vi "Error Query.vi"(8 "error in (no error)":errorcluster, 11 "VISA resource name":refnum<visa-resource-name>) -> (0 "error out":errorcluster, 1 "Error Message":string, 2 "Error Code":i32[](array[numeric]), 3 "VISA resource name out":refnum<visa-resource-name>)   [LabVIEW 2019, in "Agilent E363X Series.lvlib"]
doc: "Queries the instrument for any errors in the instrument's error queue. It will continue to read errors until all errors have been read from the instrument. Any errors will be returned in the Error Out cluster.\n\n<B>Note:</B>\nThis VI is called automatically by most driver VIs so it is not usually necessary to call this in an application."
uses:
  Agilent E363X Series.lvlib
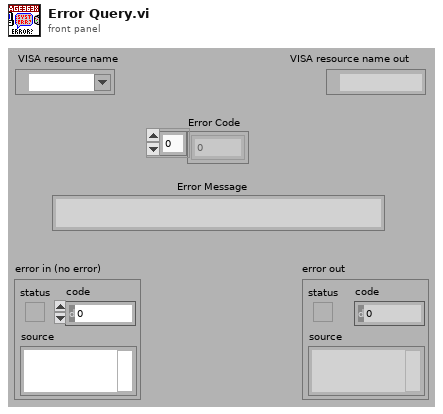
[diagram p1: front panel]
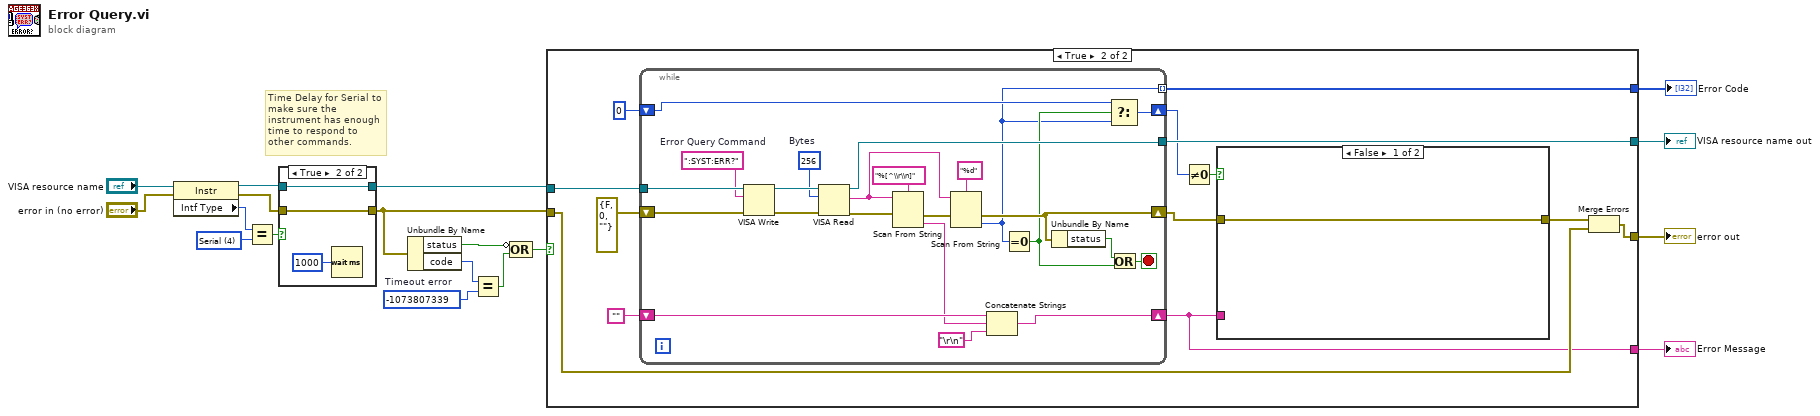
[diagram p0: block diagram]
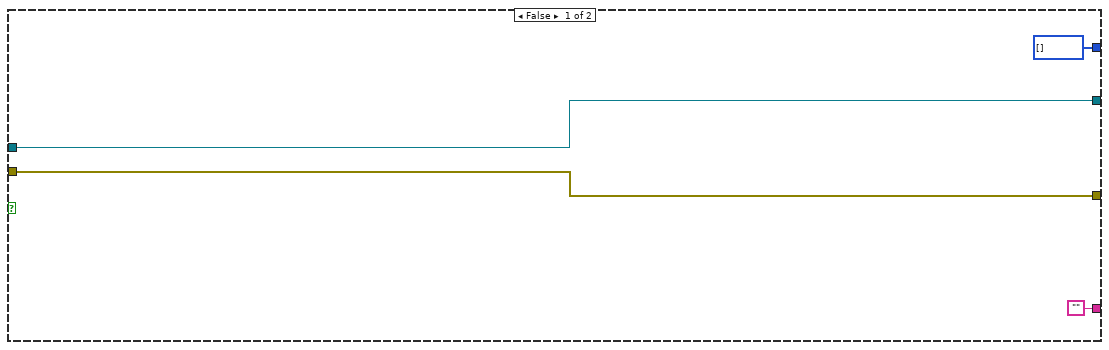
[diagram p3: hidden frame]
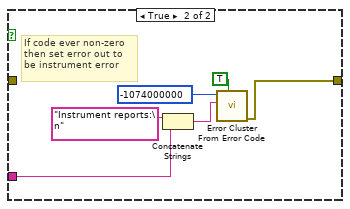
[diagram p4: hidden frame]
diagram:
  w2 = u16 4 items=["GPIB"=1, "VXI"=2, "GPIB-VXI"=3, "Serial"=4, "PXI"=5, "TCPIP"=6, "USB"=7] ("Interface Information:Interface Type")
  w15 = -1073807339  # Timeout error
  # "Time Delay for Serial to make sure the instrument has enough time to respond to other commands."
  n1 = property class="Instr"(reference="VISA resource name", error in="error in (no error)") -> (reference out=w5:refnum<visa-resource-name>, error out=w4:errorcluster, "Intf Type"=w3:u16)
  n2 = Equal?(x=w3, y=w2) -> (x = y?=w1:bool)
  n3 = case shown="True" w1 {
    tunnel: w4 -> [w19 w22]
    tunnel: [w19 w22] -> w9
    tunnel: w5 -> [w20 w21]
    tunnel: [w20 w21] -> w8
    frame False {
    }
    frame True {
      n4 = Wait (ms)(milliseconds to wait=u32 1000) -> ()  [unwired: 1 out]
    }
  }
  n5 = Unbundle By Name(w9) -> ("status"=w16:bool, "code"=w13:i32)
  n6 = Equal?(x=w13, y=w15) -> (x = y?=w14:bool)
  n7 = Compound Arithmetic op=OR(invert w16, w14) -> (w12:bool)
  n8 = case shown="True" w12 {
    tunnel: [w27 w40] -> w18
    tunnel: w8 -> [w27 w39]
    tunnel: w9 -> [w26 w33]
    tunnel: [w26 w37] -> w17
    tunnel: ["" w30] -> w11
    tunnel: [i32[] [] w29] -> w10
    frame False {
    }
    frame True {
      n9 = while {
        tunnel: [w70] -> w40
        tunnel: w39 -> [w69]
        shift-right: [w57] -> w30
        shift-left: "" -> [w60]
        shift-right: [w55] -> w31
        shift-left: 0 -> [w56]
        shift-right: [w53] -> w28
        shift-left: errorcluster {"status"=FALSE, "code"=0, "source"=""} ("error in (no error)") -> [w54]
        tunnel: [w48] -> w29 mode=indexing
        stop <- w63 stop-if-true
        w67 = u32 256  # Bytes
        w65 = ":SYST:ERR?"  # Error Query Command
        n10 = VISA Write(VISA resource name=w69, write buffer=w65, error in (no error)=w54) -> (VISA resource name out=w68:refnum<visa-resource-name>, error out=w66:errorcluster)  [unwired: 1 out]
        n11 = VISA Read(VISA resource name=w68, byte count=w67, error in (no error)=w66) -> (VISA resource name out=w70:refnum<visa-resource-name>, read buffer=w61:string, error out=w52:errorcluster)  [unwired: 1 out]
        n12 = Scan From String(format string="%[^\\r\\n]", input string=w61, error in=w52) -> (error out=w51:errorcluster, output 1=w58:string)  [unwired: 2 in, 2 out]
        n13 = Scan From String(format string="%d", input string=w61, error in=w51) -> (error out=w53:errorcluster, output 1=w48:i32)  [unwired: 2 in, 2 out]
        n14 = Concatenate Strings(w60, w58, "\r\n") -> (w57:string)
        n15 = Equal To 0?(x=w48) -> (x = 0?=w49:bool)
        n16 = Unbundle By Name(w53) -> ("status"=w50:bool)
        n17 = Select(t=w56, s=w49, f=w48) -> (s? t:f=w55:i32)
        n18 = Or(x=w50, y=w49) -> (x .or. y?=w63:bool)
      }
      n19 = Not Equal To 0?(x=w31) -> (x != 0?=w35:bool)
      n20 = case shown="False" w35 {
        tunnel: w30 -> [_ w43]
        tunnel: [w41 w42] -> w34
        tunnel: w28 -> [w41 _]
        frame False {
        }
        frame True {
          # "If code ever non-zero\nthen set error out to\nbe instrument error"
          n21 = Concatenate Strings("Instrument reports:\n" ("Source"), w43) -> (w44:string)
          n22 = call <vilib>:"Error Cluster From Error Code.vi"("show call chain? (False)"=TRUE, "error message (\"\")"=w44, "error code (0)"=-1074000000 ("Code")) -> ("error out"=w42:errorcluster)  [unwired: 6 in]
        }
      }
      n23 = Merge Errors(w34, w33) -> (w37:errorcluster)
    }
  }
  "VISA resource name out" <- w18
  "error out" <- w17
  "Error Message" <- w11
  "Error Code" <- w10
